vi "Cosine_similarity.vi"(6 "Type Y":enum16{"Array", "Sparse"}(ring), 7 "Type X":enum16{"Array", "Sparse"}(ring), 8 "error in":errorcluster caption="entrée d'erreur", 9 "Y":string[][](array[string]), 10 "X":string[][](array[string]), 11 "cosine_similarity":cluster{"dense_output":bool}={"dense_output"=TRUE}) -> (0 "error out":errorcluster caption="sortie d'erreur", 3 "Data":T1)   [LabVIEW 2020]
doc: "Compute cosine similarity between samples in X and Y.\n\nCosine similarity, or the cosine kernel, computes similarity as the normalized dot product of X and Y :\n\nK(X, Y) = <X, Y> / (||X||*||Y||)\n\nOn L2-normalized data, this function is equivalent to linear_kernel.\n\nParameters : \n\n- X : ndarray or sparse array, shape: (n_samples_X, n_features)\nInput data.\n\n- Y : ndarray or sparse array, shape: (n_samples_Y, n_features)\nInput data. If None, the output will be the pairwise similarities between all samples in X.\n\n- dense_output : boolean (optional), default True\nWhether to return dense output even when the input is sparse. If False, the output is sparse if both input arrays are sparse.\n\nReturns : \n\n- kernel matrix : array\nAn array with shape (n_samples_X, n_samples_Y)."
uses:
  Cosine_similarity.lvclass
panel:
  out "Cosine_similarity.lvclass":refnum<class "Cosine_similarity.lvclass">
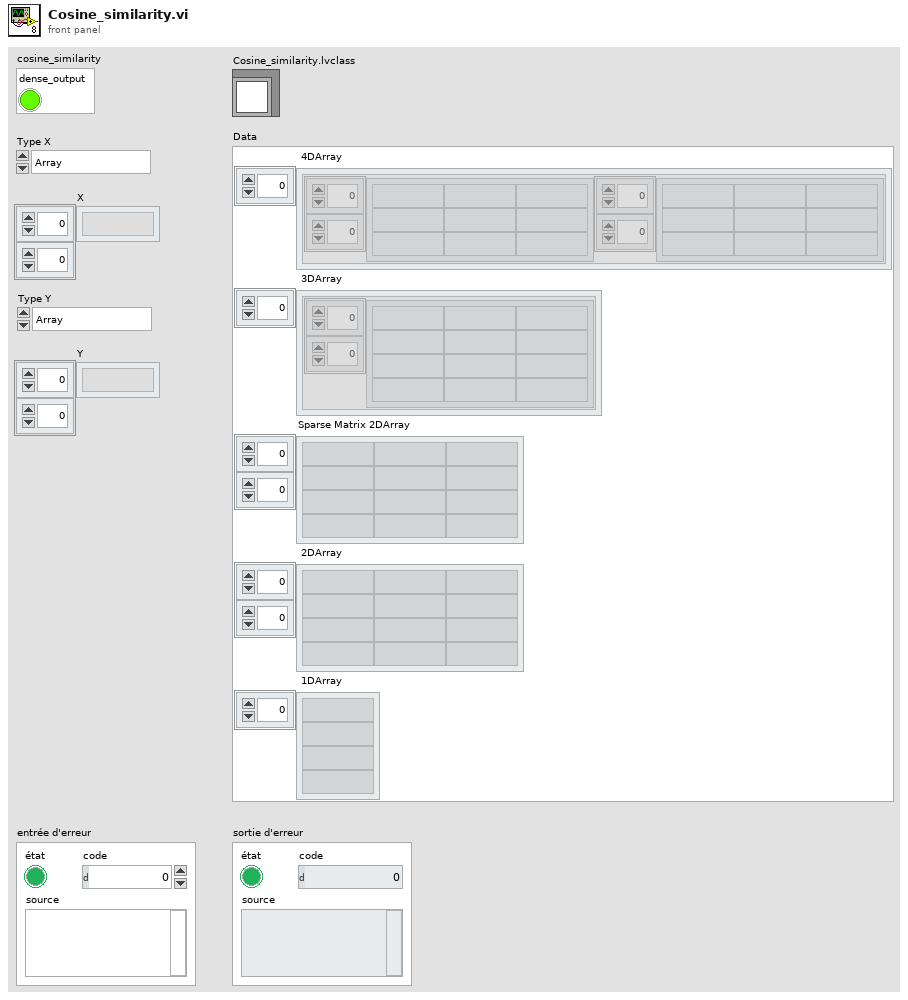
[diagram p1: front panel]
types:
  T1 = cluster{" 4DArray":cluster{"1":string[][], "2":string[][]}[], " 3DArray":cluster{"Tableau":string[][]}[], "Sparse Matrix 2DArray":string[][], " 2DArray":string[][], " 1DArray":string[]}
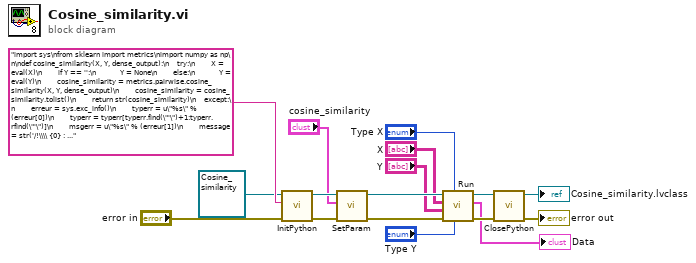
[diagram p0: block diagram]
diagram:
  n1 = call-dynamic "InitPython.vi"("error in (no error)"="error in", "Python Instruction"="import sys\nfrom sklearn import metrics\nimport numpy as np\n\ndef cosine_similarity(X, Y, dense_output):\n    try:\n        X = eval(X)\n        if Y == '':\n            Y = None\n        else:\n            Y = eval(Y)\n        cosine_similarity = metrics.pairwise.cosine_similarity(X, Y, dense_output)\n        cosine_similarity = cosine_similarity.tolist()\n        return str(cosine_similarity)\n    except:\n        erreur = sys.exc_info()\n        typerr = u\"%s\" % (erreur[0])\n        typerr = typerr[typerr.find(\"'\")+1:typerr.rfind(\"'\")]\n        msgerr = u\"%s\" % (erreur[1])\n        message = str('/!\\\\ {0} : {1}'. format(typerr,msgerr))\n        return message", "Scikit-learn en entrée"=refnum<class "Cosine_similarity.lvclass"> refnum ("Cosine_similarity.lvclass")) -> ("error out"=w10:errorcluster, "Scikit-learn en sortie"=w12:refnum<class "Cosine_similarity.lvclass">)  [unwired: 7 in]
  n2 = call-dynamic "SetParam.vi"("error in (no error)"=w10, "cosine_similarity"="cosine_similarity", "Cosine_similarity.lvclass"=w12) -> ("error out"=w8:errorcluster, "Cosine_similarity.lvclass"=w9:refnum<class "Cosine_similarity.lvclass">)  [unwired: 7 in]
  n3 = call-dynamic "Run.vi"("Type Y"="Type Y", "Type X"="Type X", "error in (no error)"=w8, "Y"="Y", "X"="X", "Cosine_similarity.lvclass"=w9) -> ("error out"=w13:errorcluster, "Data"=→"Data":T1, "Cosine_similarity.lvclass"=w14:refnum<class "Cosine_similarity.lvclass">)  [unwired: 3 in]
  n4 = call-dynamic "ClosePython.vi"("error in (no error)"=w13, "Scikit-learn en entrée"=w14) -> ("error out"=→"error out":errorcluster, "Scikit-learn en sortie"=→"Cosine_similarity.lvclass":refnum<class "Cosine_similarity.lvclass">)  [unwired: 8 in]
